vi "Periodic Tasks.vi"(8 "error in":errorcluster) -> ()   [LabVIEW 2016]
doc: "This VI runs in parallel to other tasks. It can contain as many user-defined periodic loops as you need. These can carry out PID or other sorts of timed response."
uses:
  <vilib>/Rock Robotics/WPI/Encoder/WPI_EncoderType.ctl
  <vilib>/Rock Robotics/SystemInterfaces/DIO/FPGA_DIOChannel.ctl
  <vilib>/Rock Robotics/WPI/Counter/WPI_CounterDigitalInputToDigitalSource.vi
  Encoder Rate Shooter.vi
  Encoder Distance.vi
  Ultrasonic distance.vi
  Cam X.vi
  Cam Y.vi
  Cam H.vi
  Cam W.vi
  <vilib>/Rock Robotics/WPI/Ultrasonic/WPI_SonarSRF04DigitalOpen.vi
  <vilib>/Rock Robotics/WPI/Ultrasonic/WPI_SonarSRF04DigitalGetRange.vi
  <vilib>/Rock Robotics/WPI/Ultrasonic/WPI_SonarSRF04DigitalClose.vi
panel:
  out "Height":dbl
  out "Width":dbl
  out "Y":dbl
  out "X":dbl
  in  "Average Bits":u8=3 max=15
  in  "Scaling factor (V/in)":dbl=0.0098
  in  "stop 3":bool
  out "distance":dbl(slide)=125.0 scale=0.0..250.0 scale format="%3d"
  out "Encoder Direction 2":string
  out "Encoder Alarm Status 2":string
  in  "Reset Encoder? 2":bool
  in  "stop 2":bool
  out "Encoder Distance 2":dbl
  out "Encoder Rate (distance/sec) 2":dbl
  in  "Minimum Rate 2":dbl=20.0
  in  "A Channel 2":T1=enum."DIO 2"
  in  "B Channel 2":T1=enum."DIO 3"
  in  "DistancePerCount 2":dbl=1.0
  in  "Decoding Type 2":T2=enum."4x"
  in  "Invert Direction 2":bool=TRUE
  in  "Number Samples to Average 2":u8=4 min=1 max=128
  out "Encoder Direction":string
  out "Encoder Alarm Status":string
  in  "Reset Encoder?":bool
  in  "stop":bool
  out "Encoder Distance":dbl
  out "Encoder Rate (distance/sec)":dbl
  in  "Minimum Rate":dbl=20.0
  in  "A Channel":T1
  in  "B Channel":T1=enum."DIO 1"
  in  "DistancePerCount":dbl=1.0
  in  "Decoding Type":T2=enum."4x"
  in  "Invert Direction":bool
  in  "Number Samples to Average":u8=4 min=1 max=128
  # "DO NOT INVERT"
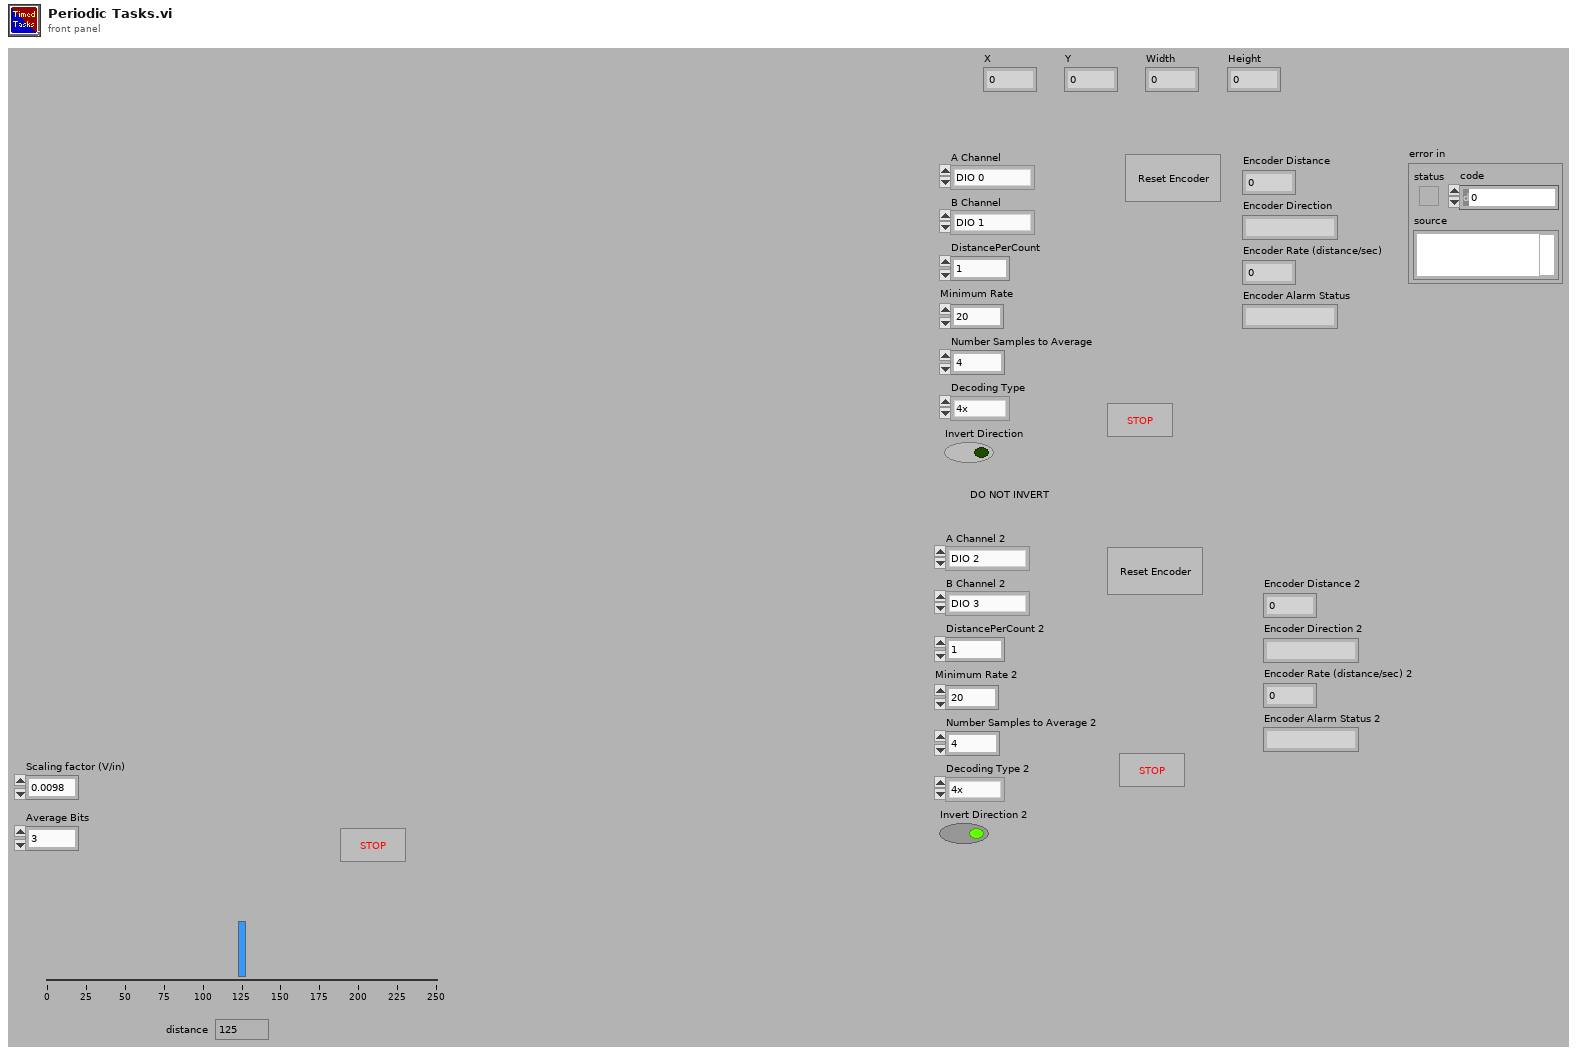
[diagram p1: front panel]
types:
  T1 = typedef "FPGA_DIOChannel.ctl" = enum8{"DIO 0", "DIO 1", "DIO 2", "DIO 3", "DIO 4", "DIO 5", "DIO 6", "DIO 7", "DIO 8", "DIO 9", "DIO MXP 0", "DIO MXP 1", "DIO MXP 2", "DIO MXP 3", "DIO MXP 4", "DIO MXP 5", "DIO MXP 6", "DIO MXP 7", "DIO MXP 8", "DIO MXP 9", "DIO MXP 10", "DIO MXP 11", "DIO MXP 12", "DIO MXP 13", "DIO MXP 14", "DIO MXP 15", "SPI Port CS1", "SPI Port CS2", "SPI Port CS3", "SPI Port MISO", "SPI Port MOSI", "Invalid"}
  T2 = typedef "WPI_EncoderType.ctl" = enum16{"1x", "2x", "4x"}
  T3 = typedef "WPI_JoystickDevRef.ctl" = cluster{"Device":T4}
  T4 = typedef "WPI_JoystickDeviceEnum.ctl" = enum16{"USB 0", "USB 1", "USB 2", "USB 3", "USB 4", "USB 5"}
  T5 = typedef "WPI_RobotDriveDevRef.ctl" = cluster{"DevStatus":errorcluster, "Motors[]":T6[], "Square Inputs":bool, "Max Output":dbl}
  T6 = typedef "WPI_MotorControlDeviceRef.ctl" = cluster{"DeviceStatus":errorcluster, "Type":T7, "PWM":cluster{"PWM Channel":T8, "DeadBand":T9}, "CAN":cluster{"Device Number":u8, "SetOutput VI Ref":variant, "GetOutput VI Ref":variant, "Enable VI Ref":variant, "Disable VI Ref":variant, "Data":variant}, "Invert":bool}
  T7 = typedef "WPI_MotorControlType.ctl" = enum16{"PWM", "CAN"}
  T8 = typedef "FPGA_DIOPWMChannel.ctl" = enum8{"PWM 0", "PWM 1", "PWM 2", "PWM 3", "PWM 4", "PWM 5", "PWM 6", "PWM 7", "PWM 8", "PWM 9", "PWM MXP 0", "PWM MXP 1", "PWM MXP 2", "PWM MXP 3", "PWM MXP 4", "PWM MXP 5", "PWM MXP 6", "PWM MXP 7", "PWM MXP 8", "PWM MXP 9", "Invalid"}
  T9 = typedef "WPI_PWMDeadband.ctl" = cluster{"Name":string, "maxPositivePwm":i32, "minPositivePwm":i32, "centerPwm":i32, "maxNegativePwm":i32, "minNegativePwm":i32, "angularRange":u16}
  T10 = cluster{"JoystickDevRef":T3, "RobotDriveDevRef":T5}
  T11 = typedef "WPI_DigitalInputDevRef.ctl" = cluster{"DevStatus":errorcluster, "DIO Channel":T1}
  T12 = typedef "WPI_UltrasonicDeviceRef.ctl" = cluster{"DevStatus":errorcluster, "Ping Channel":T1, "Echo Channel":T1, "CntIndex":T13}
  T13 = typedef "FPGA_CounterCtrSystemIndex.ctl" = enum8{"Ctr 0", "Ctr 1", "Ctr 2", "Ctr 3", "Ctr 4", "Ctr 5", "Ctr 6", "Ctr 7", "Invalid"}
  T14 = typedef "FPGA_CounterEncoderSourceConvertionLVSourceType.ctl" = cluster{"DevStatus":errorcluster, "AnalogTriggerMode?":bool, "DigitalMode":cluster{"DIO Channel":T15}, "AnalogTriggerMode":cluster{"AnalogTriggerIndex":T16, "OutputType":T17}}
  T15 = typedef "FPGA_DIODigitalSourceChannel.ctl" = enum8{"DIO 0", "DIO 1", "DIO 2", "DIO 3", "DIO 4", "DIO 5", "DIO 6", "DIO 7", "DIO 8", "DIO 9", "DIO MXP 0", "DIO MXP 1", "DIO MXP 2", "DIO MXP 3", "DIO MXP 4", "DIO MXP 5", "DIO MXP 6", "DIO MXP 7", "DIO MXP 8", "DIO MXP 9", "DIO MXP 10", "DIO MXP 11", "DIO MXP 12", "DIO MXP 13", "DIO MXP 14", "DIO MXP 15", "Disabled"}
  T16 = typedef "FPGA_AnalogTriggerIndex.ctl" = enum8{"Trig 0", "Trig 1", "Trig 2", "Trig 3", "Trig 4", "Trig 5", "Trig 6", "Trig 7", "Invalid"}
  T17 = typedef "FPGA_AnalogTriggerOutType.ctl" = enum16{"InWindow", "TriggerState", "Rising", "Falling"}
  T18 = typedef "WPI_EncoderDevRef.ctl" = cluster{"DevStatus":errorcluster, "EncoderIndex":T19, "CounterIndex":T13, "DistancePerCount":dbl, "Decoding Type":T2}
  T19 = typedef "FPGA_EncoderIdx.ctl" = enum8{"Enc 0", "Enc 1", "Enc 2", "Enc 3", "Enc 4", "Enc 5", "Enc 6", "Enc 7", "Invalid"}
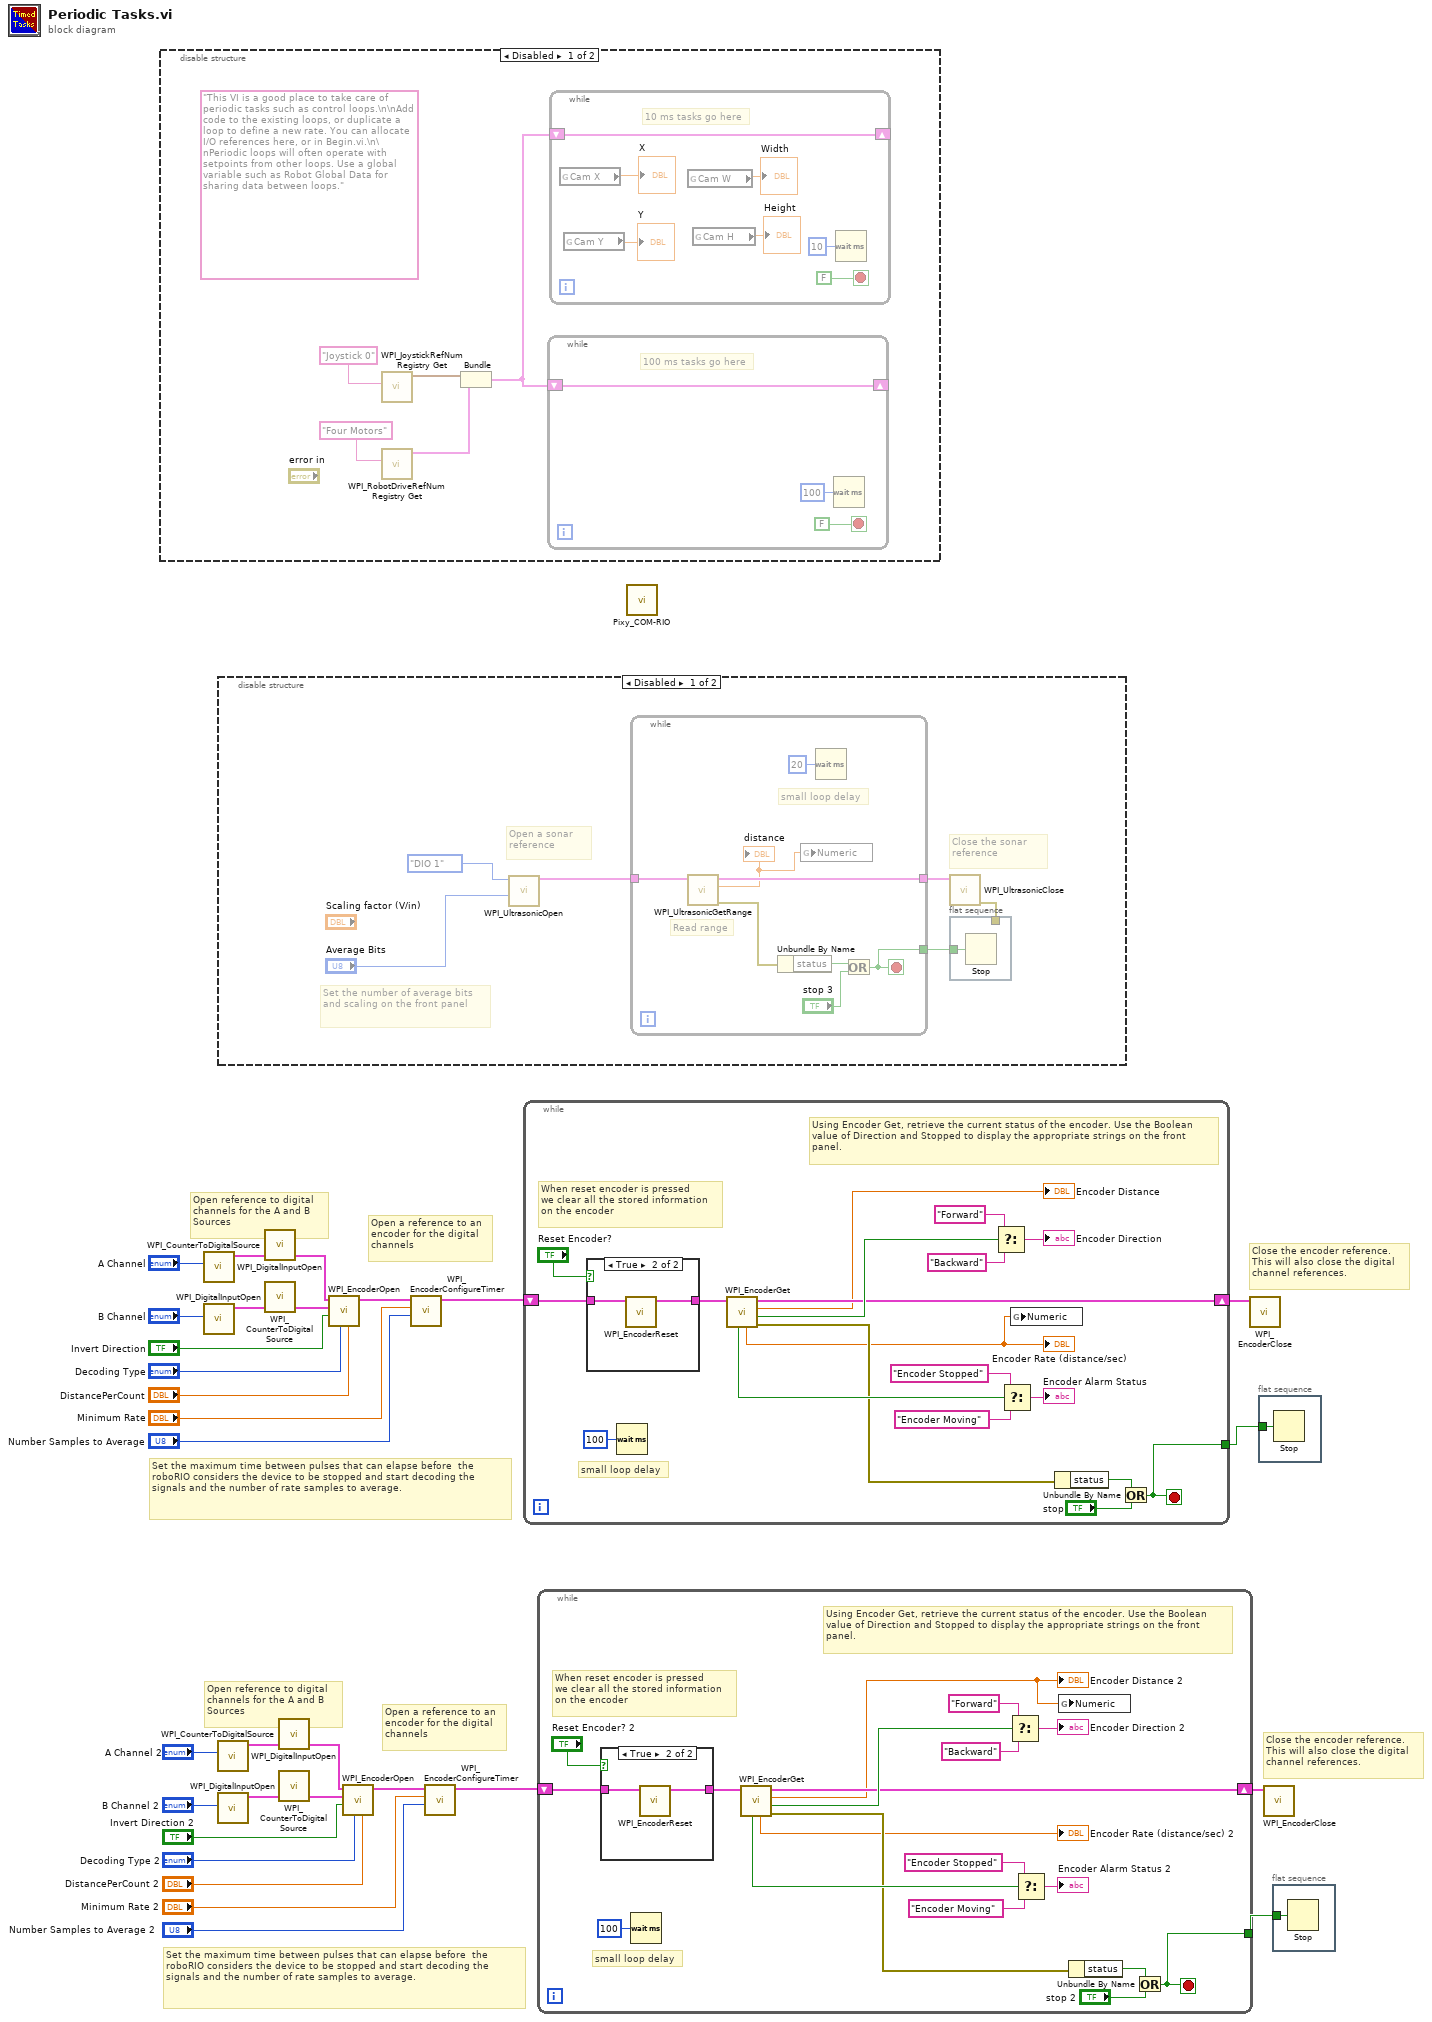
[diagram p0: block diagram]
diagram:
  # "Close the encoder reference.\nThis will also close the digital \nchannel references."
  # "Set the maximum time between pulses that can elapse before  the roboRIO considers the device to be stopped and start decoding the signals and the number of rate samples to average."
  # "Open a reference to an\nencoder for the digital \nchannels"
  # "Open reference to digital \nchannels for the A and B\nSources"
  # "Close the encoder reference.\nThis will also close the digital \nchannel references."
  # "Set the maximum time between pulses that can elapse before  the roboRIO considers the device to be stopped and start decoding the signals and the number of rate samples to average."
  # "Open a reference to an\nencoder for the digital \nchannels"
  # "Open reference to digital \nchannels for the A and B\nSources"
  n1 = disable-structure shown="Disabled" {
    frame Disabled {
      (unwired) "This VI is a good place to take care of periodic tasks such as control loops.\n\nAdd code to the existing loops, or duplicate a loop to define a new rate. You can allocate I/O references here, or in Begin.vi.\n\nPeriodic loops will often operate with setpoints from other loops. Use a global variable such as Robot Global Data for sharing data between loops."
      n2 = call <vilib>:"WPI_JoystickRefNum Registry Get.vi"("refnum name"="Joystick 0") -> ("JoystickDevRef"=w33:T3)  [unwired: 1 in, 9 out]
      n3 = call <vilib>:"WPI_RobotDriveRefNum Registry Get.vi"("refnum name"="Four Motors") -> ("RobotDriveDevRef"=w32:T5)  [unwired: 1 in, 9 out]
      n4 = Bundle("JoystickDevRef"=w33, "RobotDriveDevRef"=w32) -> (w31:T10)  [unwired: 1 out]
      n5 = while {
        shift-right: [w36] -> _
        shift-left: w31 -> [w36]
        stop <- FALSE stop-if-true
        # "100 ms tasks go here"
        n6 = Wait (ms)(milliseconds to wait=u32 100) -> ()  [unwired: 1 out]
      }
      n7 = while {
        shift-right: [w43] -> _
        shift-left: w31 -> [w43]
        stop <- FALSE stop-if-true
        # "10 ms tasks go here"
        n8 = global read "Cam X.vi" "Cam X"() -> (→"X":dbl)
        n9 = global read "Cam Y.vi" "Cam Y"() -> (→"Y":dbl)
        n10 = global read "Cam W.vi" "Cam W"() -> (→"Width":dbl)
        n11 = global read "Cam H.vi" "Cam H"() -> (→"Height":dbl)
        n12 = Wait (ms)(milliseconds to wait=u32 10) -> ()  [unwired: 1 out]
      }
    }
    frame Enabled {
    }
  }
  n13 = call <vilib>:"WPI_DigitalInputOpen.vi"("DIO Channel"="A Channel") -> ("DigitalInputDevRef"=w20:T11)  [unwired: 1 in, 9 out]
  n14 = call <vilib>:"WPI_DigitalInputOpen.vi"("DIO Channel"="B Channel") -> ("DigitalInputDevRef"=w19:T11)  [unwired: 1 in, 9 out]
  n15 = call <vilib>:"WPI_DigitalInputOpen.vi"("DIO Channel"="A Channel 2") -> ("DigitalInputDevRef"=w11:T11)  [unwired: 1 in, 9 out]
  n16 = call <vilib>:"WPI_DigitalInputOpen.vi"("DIO Channel"="B Channel 2") -> ("DigitalInputDevRef"=w12:T11)  [unwired: 1 in, 9 out]
  n17 = disable-structure shown="Disabled" {
    frame Disabled {
      # "Set the number of average bits and scaling on the front panel"
      # "Close the sonar reference"
      # "Open a sonar reference"
      n18 = call-poly <vilib>:"WPI_UltrasonicOpen.vi"("Echo DIO Channel"="Average Bits", "Ping DIO Channel"=FPGA_DIOChannel."DIO 1") -> ("SonarSRF04DevRef"=w50:T12)  [unwired: 8 in, 1 out]
      n19 = while {
        tunnel: w50 -> [w54]
        tunnel: [w60] -> w48
        tunnel: [w55] -> w51
        stop <- w55 stop-if-true
        # "small loop delay"
        # "Read range"
        n20 = call-poly <vilib>:"WPI_UltrasonicGetRange.vi"("SonarSRF04DevRef"=w54) -> ("error out"=w56:errorcluster, "Distance"=w53:dbl, "SonarSRF04DevRef"=w60:T12)  [unwired: 8 in]
        "distance" <- w53
        n21 = Unbundle By Name(w56) -> ("status"=w58:bool)
        n22 = global write "Ultrasonic distance.vi" "Numeric"(w53) -> ()
        n23 = Wait (ms)(milliseconds to wait=u32 20) -> ()  [unwired: 1 out]
        n24 = Or(x=w58, y="stop 3") -> (x .or. y?=w55:bool)
      }
      n25 = call-poly <vilib>:"WPI_UltrasonicClose.vi"("SonarSRF04DevRef"=w48) -> ("error out"=w47:errorcluster)  [unwired: 10 in]
      n26 = flat-sequence {
        tunnel: w51 -> [w52]
        tunnel: w47 -> [_]
        frame #0 {
          n27 = Stop(stop? (T)=w52) -> ()
        }
      }
    }
    frame Enabled {
    }
  }
  n28 = call-poly <vilib>:"WPI_CounterToDigitalSource.vi"("DigitalInputDevRef"=w20) -> ("Digital Source"=w21:T14)  [unwired: 6 out]
  n29 = call-poly <vilib>:"WPI_CounterToDigitalSource.vi"("DigitalInputDevRef"=w19) -> ("Digital Source"=w18:T14)  [unwired: 6 out]
  n30 = call-poly <vilib>:"WPI_CounterToDigitalSource.vi"("DigitalInputDevRef"=w11) -> ("Digital Source"=w10:T14)  [unwired: 6 out]
  n31 = call-poly <vilib>:"WPI_CounterToDigitalSource.vi"("DigitalInputDevRef"=w12) -> ("Digital Source"=w13:T14)  [unwired: 6 out]
  n32 = call <vilib>:"WPI_EncoderOpen.vi"("DistancePerCount"="DistancePerCount", "Decoding Type"="Decoding Type", "Invert Direction (False)"="Invert Direction", "BSource"=w18, "ASource"=w21) -> ("EncoderDevRef"=w28:T18)  [unwired: 3 in, 3 out]
  n33 = call <vilib>:"WPI_EncoderOpen.vi"("DistancePerCount"="DistancePerCount 2", "Decoding Type"="Decoding Type 2", "Invert Direction (False)"="Invert Direction 2", "BSource"=w13, "ASource"=w10) -> ("EncoderDevRef"=w3:T18)  [unwired: 3 in, 3 out]
  n34 = call <vilib>:"WPI_EncoderConfigureTimer.vi"("Number Samples to Average"="Number Samples to Average", "Minimum Rate"="Minimum Rate", "EncoderDevRef"=w28) -> ("EncoderDevRef"=w27:T18)  [unwired: 1 in, 7 out]
  n35 = call <vilib>:"WPI_EncoderConfigureTimer.vi"("Number Samples to Average"="Number Samples to Average 2", "Minimum Rate"="Minimum Rate 2", "EncoderDevRef"=w3) -> ("EncoderDevRef"=w4:T18)  [unwired: 1 in, 7 out]
  n36 = while {
    shift-right: [w74] -> w17
    shift-left: w27 -> [w79]
    tunnel: [w73] -> w16
    stop <- w73 stop-if-true
    # "small loop delay"
    # "Using Encoder Get, retrieve the current status of the encoder. Use the Boolean value of Direction and Stopped to display the appropriate strings on the front panel."
    # "When reset encoder is pressed\nwe clear all the stored information\non the encoder"
    n37 = case shown="True" "Reset Encoder?" {
      tunnel: w79 -> [w80 w82]
      tunnel: [w80 w81] -> w77
      frame False {
      }
      frame True {
        n38 = call <vilib>:"WPI_EncoderReset.vi"("EncoderDevRef"=w82) -> ("EncoderDevRef"=w81:T18)  [unwired: 1 in, 9 out]
      }
    }
    n39 = Wait (ms)(milliseconds to wait=u32 100) -> ()  [unwired: 1 out]
    n40 = call <vilib>:"WPI_EncoderGet.vi"("EncoderDevRef"=w77) -> ("error out"=w71:errorcluster, "Direction"=w76:bool, "Distance"=→"Encoder Distance":dbl, "EncoderDevRef"=w74:T18, "Rate"=w62:dbl, "Stopped"=w75:bool)  [unwired: 1 in, 4 out]
    "Encoder Rate (distance/sec)" <- w62
    n41 = Select(t="Forward", s=w76, f="Backward") -> (s? t:f=→"Encoder Direction":string)
    n42 = Select(t="Encoder Stopped", s=w75, f="Encoder Moving") -> (s? t:f=→"Encoder Alarm Status":string)
    n43 = global write "Encoder Rate Shooter.vi" "Numeric"(w62) -> ()
    n44 = Unbundle By Name(w71) -> ("status"=w69:bool)
    n45 = Or(x=w69, y="stop") -> (x .or. y?=w73:bool)
  }
  n46 = while {
    shift-right: [w96] -> w14
    shift-left: w4 -> [w101]
    tunnel: [w95] -> w15
    stop <- w95 stop-if-true
    # "small loop delay"
    # "Using Encoder Get, retrieve the current status of the encoder. Use the Boolean value of Direction and Stopped to display the appropriate strings on the front panel."
    # "When reset encoder is pressed\nwe clear all the stored information\non the encoder"
    n47 = case shown="True" "Reset Encoder? 2" {
      tunnel: w101 -> [w102 w104]
      tunnel: [w102 w103] -> w99
      frame False {
      }
      frame True {
        n48 = call <vilib>:"WPI_EncoderReset.vi"("EncoderDevRef"=w104) -> ("EncoderDevRef"=w103:T18)  [unwired: 1 in, 9 out]
      }
    }
    n49 = Wait (ms)(milliseconds to wait=u32 100) -> ()  [unwired: 1 out]
    n50 = call <vilib>:"WPI_EncoderGet.vi"("EncoderDevRef"=w99) -> ("error out"=w93:errorcluster, "Direction"=w98:bool, "Distance"=w83:dbl, "EncoderDevRef"=w96:T18, "Rate"=→"Encoder Rate (distance/sec) 2":dbl, "Stopped"=w97:bool)  [unwired: 1 in, 4 out]
    "Encoder Distance 2" <- w83
    n51 = Select(t="Forward", s=w98, f="Backward") -> (s? t:f=→"Encoder Direction 2":string)
    n52 = Select(t="Encoder Stopped", s=w97, f="Encoder Moving") -> (s? t:f=→"Encoder Alarm Status 2":string)
    n53 = global write "Encoder Distance.vi" "Numeric"(w83) -> ()
    n54 = Unbundle By Name(w93) -> ("status"=w91:bool)
    n55 = Or(x=w91, y="stop 2") -> (x .or. y?=w95:bool)
  }
  n56 = call "Pixy_COM-RIO.vi"() -> ()  [unwired: 7 in, 5 out]
  n57 = call <vilib>:"WPI_EncoderClose.vi"("EncoderDevRef"=w17) -> ()  [unwired: 2 in, 9 out]
  n58 = flat-sequence {
    tunnel: w16 -> [w105]
    frame #0 {
      n59 = Stop(stop? (T)=w105) -> ()
    }
  }
  n60 = call <vilib>:"WPI_EncoderClose.vi"("EncoderDevRef"=w14) -> ()  [unwired: 2 in, 9 out]
  n61 = flat-sequence {
    tunnel: w15 -> [w106]
    frame #0 {
      n62 = Stop(stop? (T)=w106) -> ()
    }
  }
